vi "user-button.vi"() -> ()   [LabVIEW 2018]
panel:
  out "User Button":bool
  in  "stop":bool
  # "Simple example only to have a quick start.\nRun it, and then simply press the User Button in the roboRIO.\nThe LED in this panel should light up when you press the button.\n\nTo finish, click STOP."
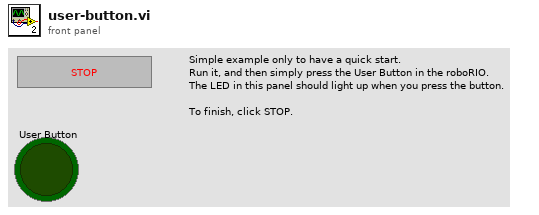
[diagram p1: front panel]
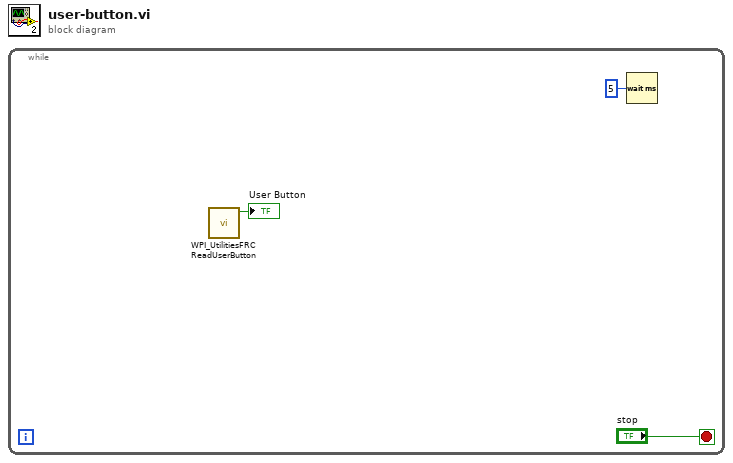
[diagram p0: block diagram]
diagram:
  n1 = while {
    stop <- "stop" stop-if-true
    n2 = call <vilib>:"WPI_UtilitiesFRC ReadUserButton.vi"() -> ("User Button"=→"User Button":bool)  [unwired: 10 in, 1 out]
    n3 = Wait (ms)(milliseconds to wait=u32 5) -> ()  [unwired: 1 out]
  }
